vi "Simulate Send DAQ Trigger.vi"(8 "error in (no error)":errorcluster, 11 "# of Triggers":i32=10) -> (0 "error out":errorcluster, 2 "# of Triggers Sent":i32, 3 "Position vs Trigger":cluster{dbl[], dbl[]}[](graph))   [LabVIEW 2019]
uses:
  Trigger State.ctl
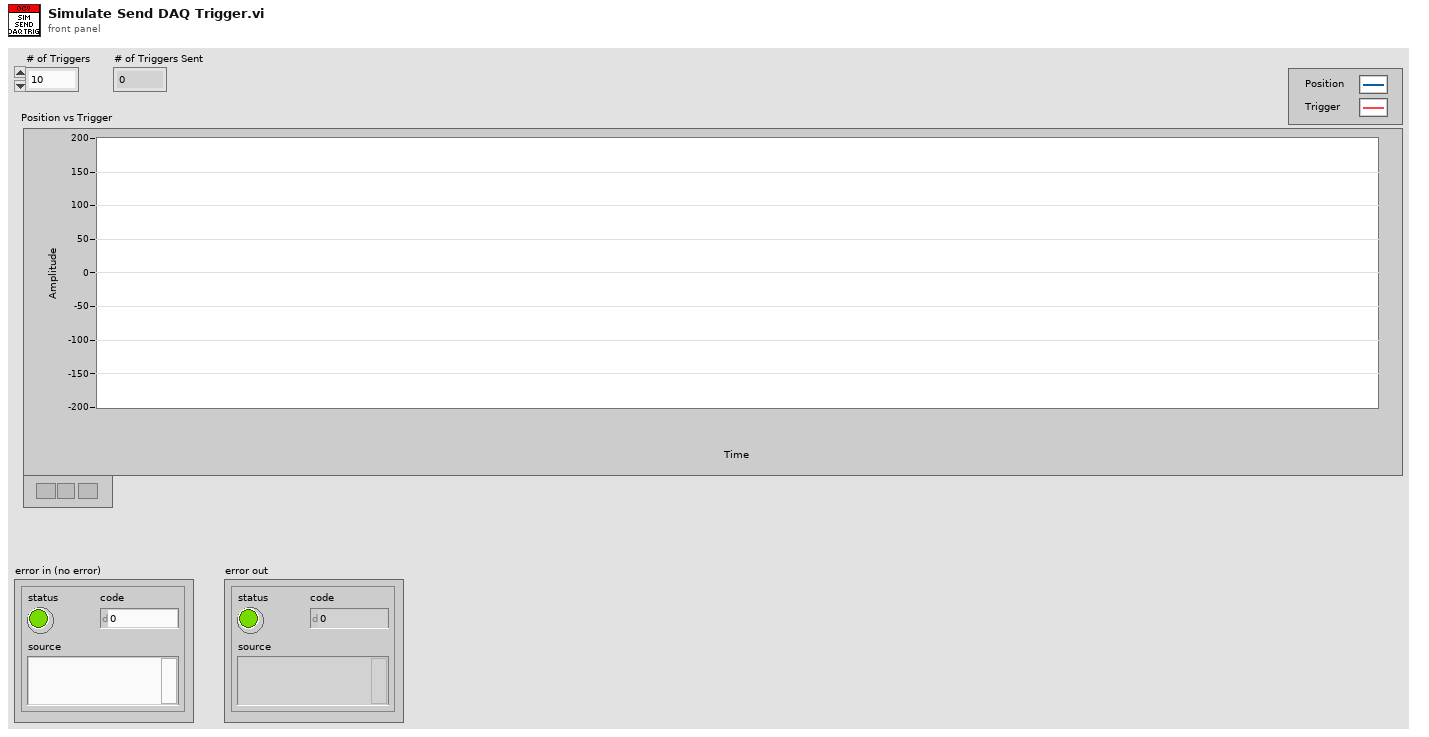
[diagram p1: front panel]
types:
  T1 = typedef "Trigger State.ctl" = enum16{"Below Threshold?", "At or Above Threshold?", "Send Trigger"}
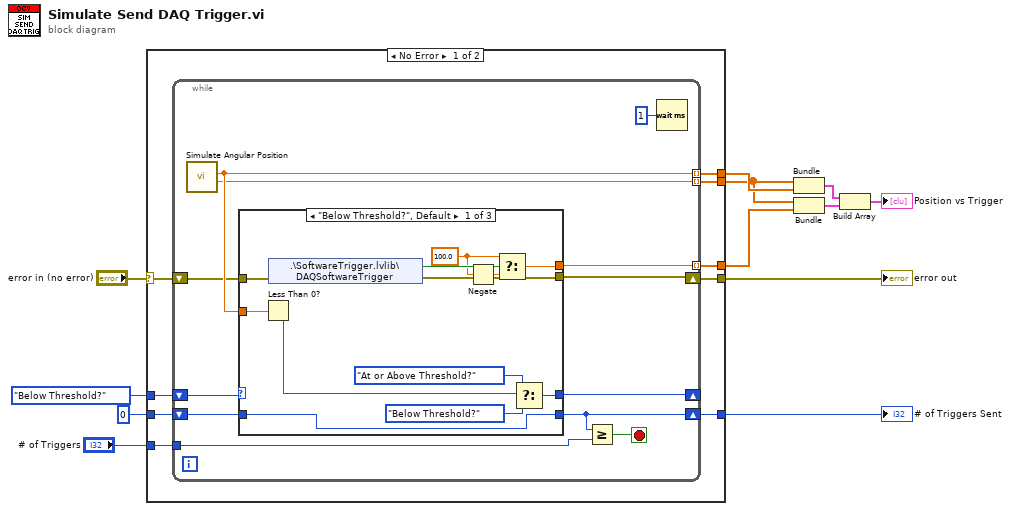
[diagram p0: block diagram]
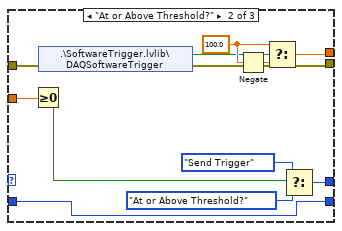
[diagram p2: hidden frame]
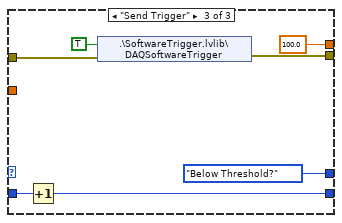
[diagram p3: hidden frame]
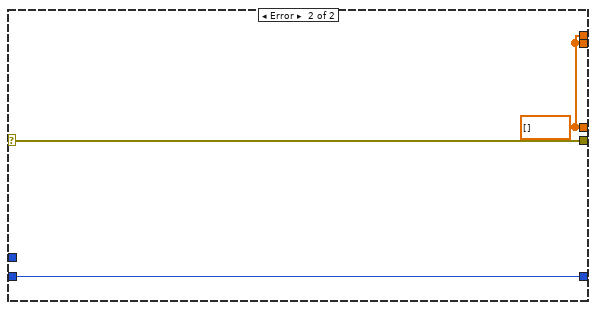
[diagram p4: hidden frame]
diagram:
  n1 = case shown="No Error" "error in (no error)" {
    selector: "error in (no error)" -> [w13 w67]
    tunnel: [w21 w66] -> w12
    tunnel: "# of Triggers" -> [w20 _]
    tunnel: 0 -> [w19 w66]
    tunnel: [w18 w67] -> w9
    tunnel: [w17 w65] -> w8
    tunnel: [w16 w65] -> w7
    tunnel: [w15 w65] -> w6
    tunnel: Trigger_State."Below Threshold?" -> [w14 _]
    frame No Error {
      n2 = while {
        shift-right: [w31] -> _
        shift-left: w14 -> [w32]
        tunnel: [w26] -> w15 mode=indexing
        tunnel: [w30] -> w17 mode=indexing
        tunnel: [w29] -> w16 mode=indexing
        shift-right: [w27] -> w18
        shift-left: w13 -> [w28]
        shift-right: [w22] -> w21
        shift-left: w19 -> [w25]
        tunnel: w20 -> [w23]
        stop <- w24 stop-if-true
        n3 = call "Simulate Angular Position.vi"() -> ("Present (s)"=w29:dbl, "Gauge"=w30:dbl)  [unwired: 10 in]
        n4 = case shown="\"Below Threshold?\", Default" w32 {
          tunnel: w30 -> [w45 w57 _]
          tunnel: [w41 w53 Trigger_State."Below Threshold?" ("t")] -> w31
          tunnel: w28 -> [w39 w50 w62]
          tunnel: [w35 w48 w61] -> w27
          tunnel: [w36 w49 100.0] -> w26
          tunnel: w25 -> [w34 w46 w59]
          tunnel: [w34 w46 w58] -> w22
          frame "Below Threshold?", Default {
            w37 = 100.0
            n5 = Less Than 0?(x=w45) -> (x < 0?=w44:bool)
            n6 = shared-variable ".\\SoftwareTrigger.lvlib\\DAQSoftwareTrigger"(error in=w39) -> (w40:bool, error out=w35:errorcluster)
            n7 = Negate(x=w37) -> (-x=w38:dbl)
            n8 = Select(t=w37, s=w40, f=w38) -> (s? t:f=w36:dbl)
            n9 = Select(t=Trigger_State."At or Above Threshold?", s=w44, f=Trigger_State."Below Threshold?") -> (s? t:f=w41:T1)
          }
          frame "At or Above Threshold?" {
            w51 = 100.0
            n10 = Greater Or Equal To 0?(x=w57) -> (x >= 0?=w56:bool)
            n11 = shared-variable ".\\SoftwareTrigger.lvlib\\DAQSoftwareTrigger"(error in=w50) -> (w47:bool, error out=w48:errorcluster)
            n12 = Negate(x=w51) -> (-x=w52:dbl)
            n13 = Select(t=w51, s=w47, f=w52) -> (s? t:f=w49:dbl)
            n14 = Select(t=Trigger_State."Send Trigger", s=w56, f=Trigger_State."At or Above Threshold?") -> (s? t:f=w53:T1)
          }
          frame "Send Trigger" {
            n15 = Increment(x=w59) -> (x+1=w58:i32)
            n16 = shared-variable ".\\SoftwareTrigger.lvlib\\DAQSoftwareTrigger"(TRUE ("Software Trigger"), error in=w62) -> (error out=w61:errorcluster)
          }
        }
        n17 = Greater Or Equal?(x=w22, y=w23) -> (x >= y?=w24:bool)
        n18 = Wait (ms)(milliseconds to wait=u32 1) -> ()  [unwired: 1 out]
      }
    }
    frame Error {
      w65 = dbl[] []
    }
  }
  "# of Triggers Sent" <- w12
  "error out" <- w9
  n19 = Bundle(w7, w8) -> (w5:cluster{dbl[], dbl[]})  [unwired: 1 in]
  n20 = Bundle(w7, w6) -> (w3:cluster{dbl[], dbl[]})  [unwired: 1 in]
  n21 = Build Array(w5, w3) -> (→"Position vs Trigger":cluster{dbl[], dbl[]}[])
